vi "ZCAN_SetRecvMerge.vi"(0 "device_handle":u32, 1 "can通道":i32, 2 "Enable":i32=1, 3 "error in (no error)":errorcluster caption="错误输入（无错误）") -> (8 "enable_success?":bool, 10 "error out":errorcluster caption="错误输出")   [LabVIEW 2020, in "zlgcan.lvlib"]
uses:
  zlgcan.lvlib
  bin/zlgcan_wrap.dll
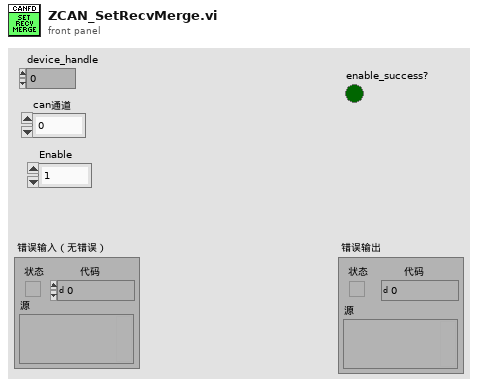
[diagram p1: front panel]
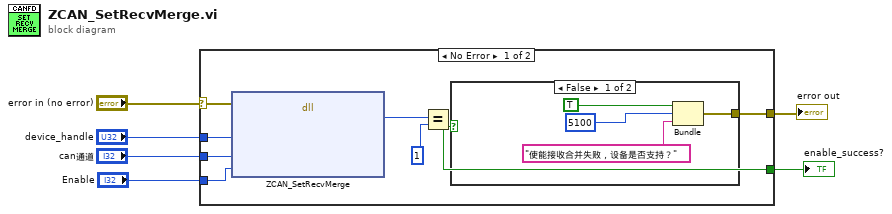
[diagram p0: block diagram]
diagram:
  n1 = case shown="No Error" "error in (no error)" {
    selector: "error in (no error)" -> [w9 w19]
    tunnel: [w12 w19] -> w5
    tunnel: "device_handle" -> [w14 _]
    tunnel: [w10 _] -> w3
    tunnel: "can通道" -> [w8 _]
    tunnel: "Enable" -> [w7 _]
    frame No Error {
      n2 = dll-call lib="E:/Jabil tools/JabilTestLib/LV/ZLG_CANFD/bin/zlgcan_wrap.dll" fn="ZCAN_SetRecvMerge" ("ZCAN_StartCAN")(error in=w9, "device_handle"=w14, "can通道"=w8, "使能"=w7) -> ("return"=w11:u32)  [unwired: 5 in, 2 out]
      n3 = Equal?(x=w11, y=1) -> (x = y?=w10:bool)
      n4 = case shown="False" w10 {
        tunnel: [w15 _] -> w12
        frame False {
          n5 = Bundle("status"=TRUE, "code"=5100, "消息"="使能接收合并失败，设备是否支持？") -> (w15:cluster{"status":bool, "code":i32, "消息":string})  [unwired: 1 in]
        }
        frame True {
        }
      }
    }
    frame Error {
    }
  }
  "error out" <- w5
  "enable_success?" <- w3
